vi "Test Basic Datatype.vi"(8 "error in (no error)":errorcluster) -> (0 "error out":errorcluster)   [LabVIEW 2018, in "JSON to LVConstant Test.lvlib"]
uses:
  JSON to LVConstant Test.lvlib
  <vilib>/JDP Science/JSONtext/JSON Value Type.ctl
  <vilib>/JDP Science/JSONtext/JSONtext.lvlib
  <vilib>/addons/_JKI Toolkits/Caraya/classes/Test/Test.lvclass
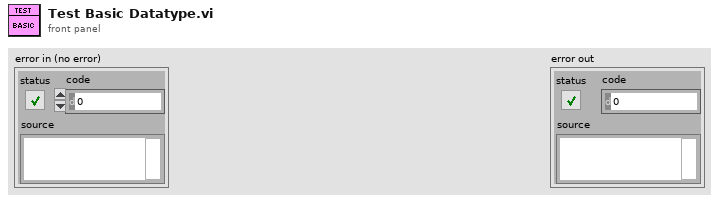
[diagram p1: front panel]
types:
  T1 = typedef "JSONtext.lvlib/JSON Value Type.ctl" = enum16{"Not a JSON Value", "JSON Object", "JSON Array", "String", "Number", "true", "false", "null"}
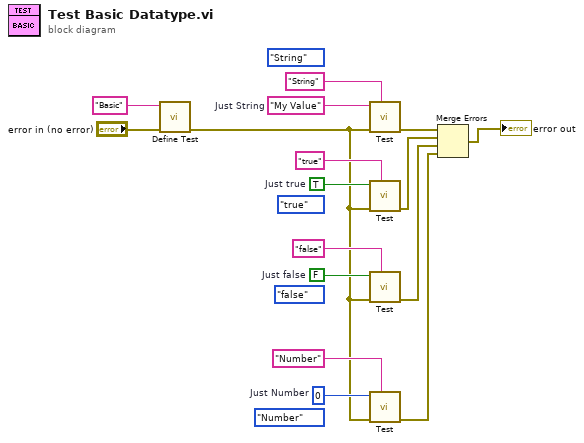
[diagram p0: block diagram]
diagram:
  (unwired) JSON_Value_Type."Number" ("JSON Value Type")
  w4 = 0  # Just Number
  (unwired) JSON_Value_Type."false" ("JSON Value Type")
  w6 = FALSE  # Just false
  (unwired) JSON_Value_Type."true" ("JSON Value Type")
  (unwired) JSON_Value_Type."String" ("JSON Value Type")
  w10 = TRUE  # Just true
  w15 = "My Value"  # Just String
  n1 = call <vilib>:"Define Test.vi"("error in (no error)"="error in (no error)", "Label (VI Title)"="Basic") -> ("error out"=w2:errorcluster)  [unwired: 9 in]
  n2 = call "Test.vi"("Label (VI Title)"="String", "error in (no error)"=w2, "Type"=w15) -> ("error out"=w14:errorcluster)  [unwired: 8 in]
  n3 = call "Test.vi"("Label (VI Title)"="true", "error in (no error)"=w2, "Type"=w10) -> ("error out"=w11:errorcluster)  [unwired: 8 in]
  n4 = call "Test.vi"("Label (VI Title)"="false", "error in (no error)"=w2, "Type"=w6) -> ("error out"=w9:errorcluster)  [unwired: 8 in]
  n5 = call "Test.vi"("Label (VI Title)"="Number", "error in (no error)"=w2, "Type"=w4) -> ("error out"=w8:errorcluster)  [unwired: 8 in]
  n6 = Merge Errors(w14, w11, w9, w8) -> (→"error out":errorcluster)
